vi "Test Compare Equal Clusters.vi"(8 "error in (no error)":errorcluster, 11 "Comparison Test Double in":refnum<class "Comparison Test Double.lvclass">) -> (0 "error out":errorcluster, 3 "Comparison Test Double out":refnum<class "Comparison Test Double.lvclass">)   [LabVIEW 2020, in "Comparison Test Double.lvclass"]
uses:
  Comparison Test Double.lvclass
  Comparison Test Double.lvclass/Comparison Test Double.ctl
  23615402-9b1f-4bd5-97a8-ca362d09ae43.vi
  C:/git/astemes-lunit/source/API/LUnit Test Case/LUnit Test Case.lvclass
  C:/git/astemes-lunit/source/Core/Runnable/Runnable.lvclass
  C:/git/astemes-lunit/tests/Comparison Test Double/Comparison Test Double.lvclass
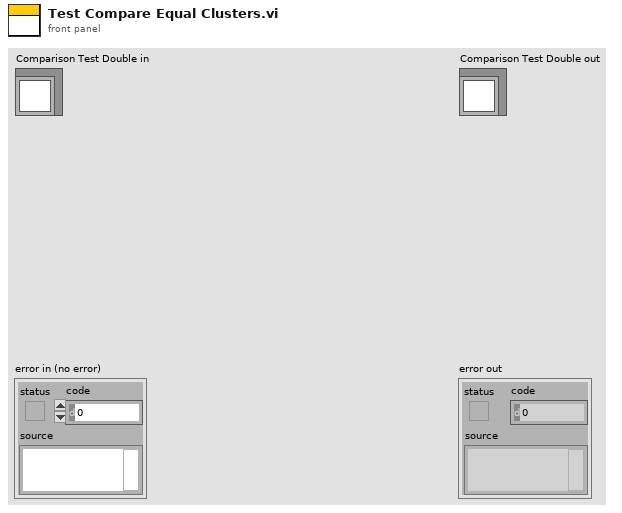
[diagram p1: front panel]
types:
  T1 = cluster{enum16{"Item A", "Item B"}, "Description":string, i32}
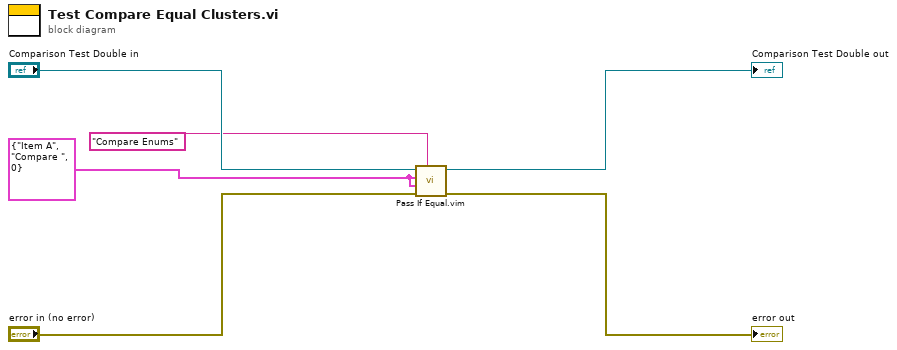
[diagram p0: block diagram]
diagram:
  w2 = T1 {enum."Item A", "Description"="Compare ", 0}
  n1 = call "Pass If Equal.vim"("Description"="Compare Enums", "error in (no error)"="error in (no error)", "Actual"=w2, "Expected"=w2, "LUnit Test Case In"="Comparison Test Double in") -> ("error out"=→"error out":errorcluster, "LUnit Test Case Out"=→"Comparison Test Double out":refnum<class "Comparison Test Double.lvclass">)  [unwired: 5 in]
